vi "NiFPGA Read - U32.vi"(8 "error in (no error)":errorcluster, 10 "Indicator":u32, 11 "Session":u32) -> (0 "error out":errorcluster, 1 "Value":u32, 3 "Session Out":u32)   [LabVIEW 2010, in "FPGA Interface Wrapper.lvlib"]
doc: "Reads an unsigned 32-bit integer value from a given indicator or control."
uses:
  <userlib>/_FPGA Interface Advanced Tools/FPGA Interface Wrapper/FPGA Interface Wrapper.lvlib
  NiFpga.dll
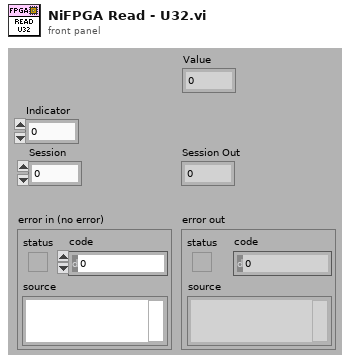
[diagram p1: front panel]
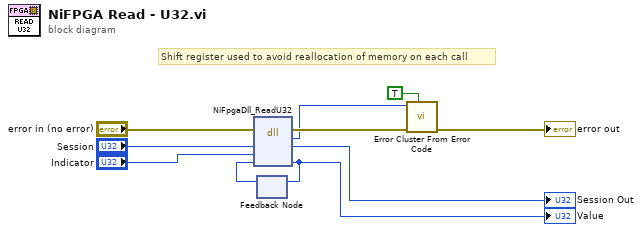
[diagram p0: block diagram]
diagram:
  # "Shift register used to avoid reallocation of memory on each call"
  n1 = feedback #1() -> (w4:u32)  [unwired: 1 in]
  n2 = dll-call lib="NiFpga.dll" fn="NiFpgaDll_ReadU32"(error in="error in (no error)", "Session"="Session", "Indicator"="Indicator", "Value"=w4) -> (error out=w2:errorcluster, "Status"=w1:i32, "Session"=→"Session Out":u32, "Value"=w5:u32)  [unwired: 3 in, 1 out]
  "Value" <- w5
  n3 = feedback-in #1(w5) -> ()
  n4 = call <vilib>:"Error Cluster From Error Code.vi"("show call chain? (False)"=TRUE, "error in (no error)"=w2, "error code (0)"=w1) -> ("error out"=→"error out":errorcluster)  [unwired: 6 in]
